vi "Parse PTR Record.vi"(8 "error in (no error)":errorcluster, 11 "STDF.lvlib:PTR":refnum<class "PTR.lvclass">) -> (0 "error out":errorcluster, 3 "PTR Data":T1)   [LabVIEW 2018, in "STDF File Parser.lvclass"]
uses:
  STDF File Parser.lvclass
  <userlib>/STDF/PTR/PTR.lvclass
  Typedefs/PTR Data.ctl
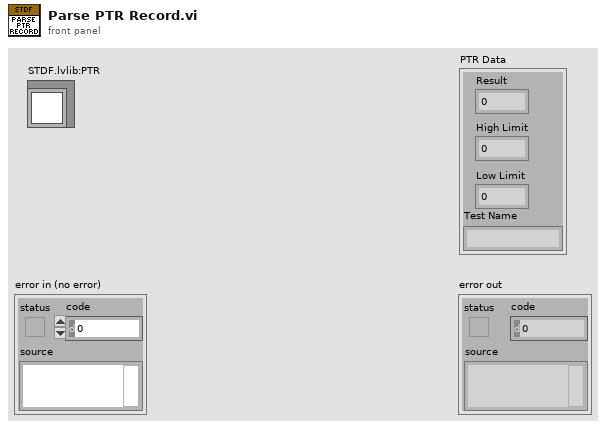
[diagram p1: front panel]
types:
  T1 = typedef "STDF File Parser.lvclass/PTR Data.ctl" = cluster{"Result":dbl, "High Limit":dbl, "Low Limit":dbl, "Test Name":string}
  T2 = typedef "STDF.lvlib/Scales and formats.ctl" = cluster{"RES_SCAL":i8, "LLM_SCAL":i8, "HLM_SCAL":i8, "UNITS":string, "C_RESFMT":string, "C_LLMFMT":string, "C_HLMFMT":string}
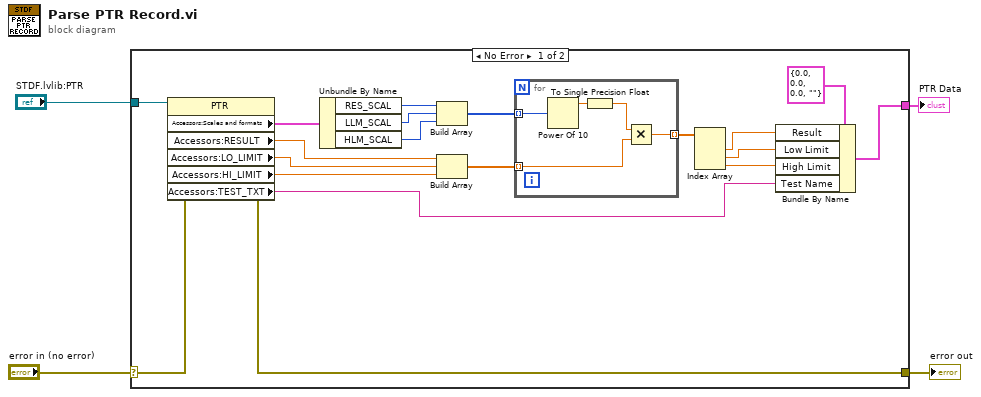
[diagram p0: block diagram]
diagram:
  n1 = case shown="No Error" "error in (no error)" {
    selector: "error in (no error)" -> [w6 w29]
    tunnel: [w5 w29] -> w3
    tunnel: "STDF.lvlib:PTR" -> [w23 _]
    tunnel: [w7 _] -> w1
    frame No Error {
      n2 = property class="PTR"(reference=w23, error in=w6) -> (error out=w5:errorcluster, "Accessors:Scales and formats"=w22:T2, "Accessors:RESULT"=w17:sgl, "Accessors:LO_LIMIT"=w16:sgl, "Accessors:HI_LIMIT"=w15:sgl, "Accessors:TEST_TXT"=w8:string)  [unwired: 1 out]
      n3 = Unbundle By Name(w22) -> ("RES_SCAL"=w21:i8, "LLM_SCAL"=w20:i8, "HLM_SCAL"=w19:i8)
      n4 = Build Array(w21, w20, w19) -> (w18:i8[])
      n5 = Build Array(w17, w16, w15) -> (w14:sgl[])
      n6 = for {
        tunnel: w18 -> [w27] mode=indexing
        tunnel: w14 -> [w25] mode=indexing
        tunnel: [w24] -> w12 mode=indexing
        n7 = Power Of 10(x=w27) -> (10^x=w28:dbl)
        n8 = To Single Precision Float(number=w28) -> (single precision float=w26:sgl)
        n9 = Multiply(x=w26, y=w25) -> (x*y=w24:sgl)
      }
      n10 = Index Array(array=w12) -> (element #1=w11:sgl, element #2=w10:sgl, element #3=w9:sgl)  [unwired: 3 in]
      n11 = Bundle By Name(cluster=T1 {"Result"=0.0, "High Limit"=0.0, "Low Limit"=0.0, "Test Name"=""} ("PTR Data"), "Result"=w11, "Low Limit"=w10, "High Limit"=w9, "Test Name"=w8) -> (w7:T1)
    }
    frame Error {
    }
  }
  "error out" <- w3
  "PTR Data" <- w1
